vi "AverageXYZ (SubVI).vi"(8 "array":dbl[][][](array[numeric])) -> (0 "Bottom uncertainty":dbl[][](array[numeric]), 1 "Bottom averages":dbl[][](array[numeric]), 2 "Top uncertainty":dbl[][](array[numeric]), 3 "Top averages":dbl[][](array[numeric]))   [LabVIEW 2016]
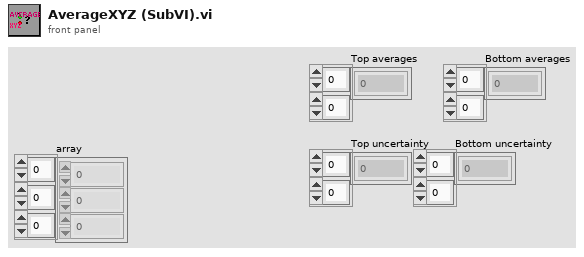
[diagram p1: front panel]
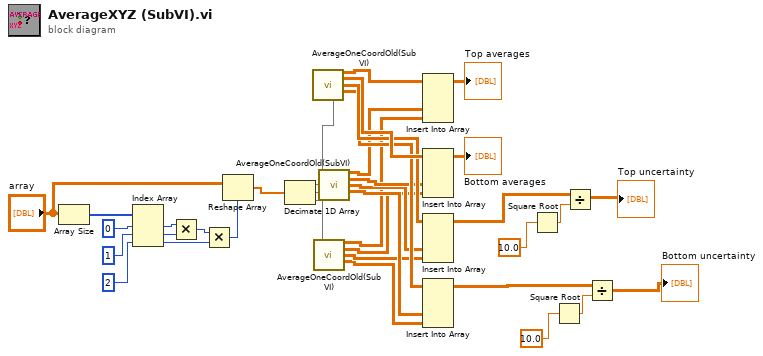
[diagram p0: block diagram]
diagram:
  n1 = Array Size(array="array") -> (size(s)=w36:i32[])
  n2 = Index Array(array=w36, index #1=0 ("index"), index #2=1 ("index"), index #3=2 ("index")) -> (element #1=w32:i32, element #2=w31:i32, element #3=w29:i32)
  n3 = Multiply(x=w32, y=w31) -> (x*y=w30:i32)
  n4 = Multiply(x=w30, y=w29) -> (x*y=w27:i32)
  n5 = Reshape Array("array", w27) -> (w26:dbl[])
  n6 = Decimate 1D Array(w26) -> (w23:dbl[], w18:dbl[], w13:dbl[])
  n7 = call "AverageOneCoordOld(SubVI).vi"("Array"=w23) -> ("Top averages"=w22:dbl[][], "Bottom averages"=w21:dbl[][], "Top SD"=w20:dbl[][], "Bottom SD"=w19:dbl[][])  [unwired: 11 in]
  n8 = call "AverageOneCoordOld(SubVI).vi"("Array"=w13) -> ("Top averages"=w12:dbl[][], "Bottom averages"=w11:dbl[][], "Top SD"=w10:dbl[][], "Bottom SD"=w9:dbl[][])  [unwired: 11 in]
  n9 = call "AverageOneCoordOld(SubVI).vi"("Array"=w18) -> ("Top averages"=w17:dbl[][], "Bottom averages"=w15:dbl[][], "Top SD"=w14:dbl[][], "Bottom SD"=w16:dbl[][])  [unwired: 11 in]
  n10 = Insert Into Array(array=w22, new element #1=w17, new element #2=w12) -> (→"Top averages":dbl[][])  [unwired: 2 in]
  n11 = Insert Into Array(array=w21, new element #1=w15, new element #2=w11) -> (→"Bottom averages":dbl[][])  [unwired: 2 in]
  n12 = Insert Into Array(array=w20, new element #1=w14, new element #2=w10) -> (w8:dbl[][])  [unwired: 2 in]
  n13 = Insert Into Array(array=w19, new element #1=w16, new element #2=w9) -> (w2:dbl[][])  [unwired: 2 in]
  n14 = Square Root(x=10.0) -> (sqrt(x)=w5:dbl)
  n15 = Square Root(x=10.0) -> (sqrt(x)=w3:dbl)
  n16 = Divide(x=w8, y=w5) -> (x/y=→"Top uncertainty":dbl[][])
  n17 = Divide(x=w2, y=w3) -> (x/y=→"Bottom uncertainty":dbl[][])
